vi "GetVelocity(rps).vi"(7 "Units":enum16{"r/s", "r/m"}(ring), 8 "error in (no error)":errorcluster, 11 "Motor Base in":refnum<class "Motor Base.lvclass">) -> (0 "error out":errorcluster, 2 "rps":dbl, 3 "Motor Base out":refnum<class "Motor Base.lvclass">)   [LabVIEW 2016, in "Motor Base.lvlib" / "Motor Base.lvclass"]
uses:
  Motor Base.lvclass
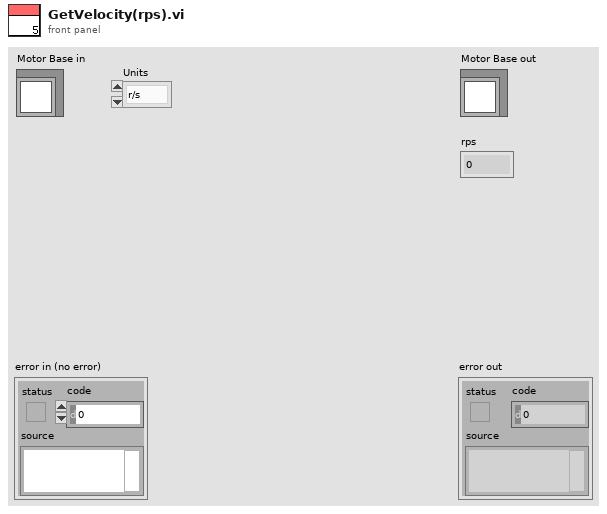
[diagram p1: front panel]
types:
  T1 = cluster{"Modes of operation":i8, "Feed(pulse)":u32, "Max motor speed(r/min)":u32, "Max torque(0.1%)":u16, "Min position limit(pulse)":i32, "Max position limit(pulse)":i32}
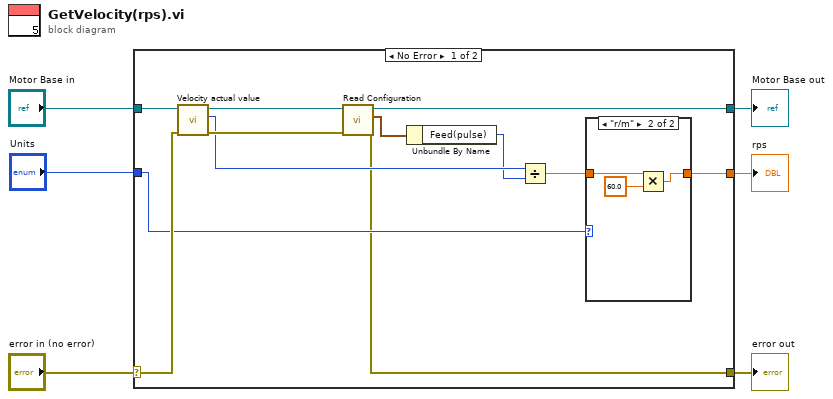
[diagram p0: block diagram]
diagram:
  n1 = case shown="No Error" "error in (no error)" {
    selector: "error in (no error)" -> [w15 w24]
    tunnel: [w7 w24] -> w5
    tunnel: [w8 w23] -> w3
    tunnel: "Motor Base in" -> [w18 w23]
    tunnel: "Units" -> [w11 _]
    tunnel: [w9 _] -> w1
    frame No Error {
      n2 = call-dynamic "Velocity actual value.vi"("error in"=w15, "Motor Base in"=w18) -> ("error out"=w17:errorcluster, "Data"=w13:i32, "Motor Base out"=w16:refnum<class "Motor Base.lvclass">)  [unwired: 7 in]
      n3 = call-dynamic "Read Configuration.vi"("error in (no error)"=w17, "Motor Base in"=w16) -> ("error out"=w7:errorcluster, "Configuration"=w14:T1, "Motor Base out"=w8:refnum<class "Motor Base.lvclass">)  [unwired: 7 in]
      n4 = Unbundle By Name(w14) -> ("Feed(pulse)"=w12:u32)
      n5 = Divide(x=w13, y=w12) -> (x/y=w10:dbl)
      n6 = case shown="\"r/m\"" w11 {
        tunnel: w10 -> [w19 w22]
        tunnel: [w19 w20] -> w9
        frame "r/s", Default {
        }
        frame "r/m" {
          n7 = Multiply(x=w22, y=60.0) -> (x*y=w20:dbl)
        }
      }
    }
    frame Error {
    }
  }
  "error out" <- w5
  "Motor Base out" <- w3
  "rps" <- w1
